vi "Load Zoom FOV table.vi"(8 "error in":errorcluster, 10 "Max Zoom":i32) -> (0 "error out":errorcluster, 2 "FOVs":dbl[][](array[numeric]))   [LabVIEW 2012, in "Sciscan Scope Daemon.lvlib"]
uses:
  Sciscan Scope Daemon.lvlib
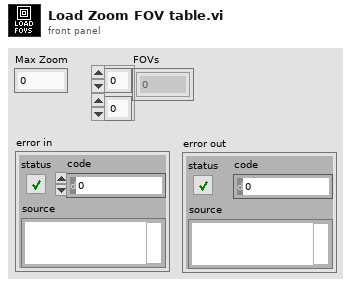
[diagram p1: front panel]
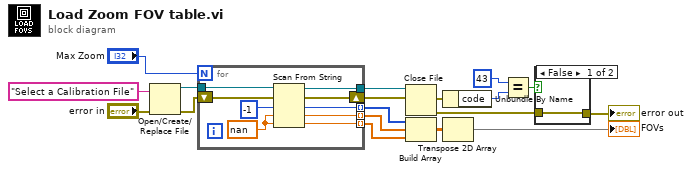
[diagram p0: block diagram]
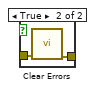
[diagram p2: hidden frame]
diagram:
  n1 = Open/Create/Replace File(error in="error in", prompt="Select a Calibration File") -> (refnum out=w17:refnum<file>, error out=w15:errorcluster)  [unwired: 4 in, 1 out]
  n2 = for {
    N: "Max Zoom" -> [_]
    tunnel: w17 -> [w26]
    tunnel: [w23] -> w16
    shift-right: [w21] -> w14
    shift-left: w15 -> [w22]
    tunnel: [w20] -> w13 mode=indexing
    tunnel: [w19] -> w12 mode=indexing
    tunnel: [w18] -> w9 mode=indexing
    w24 = nan ("input 3")
    n3 = Scan From String(w26, w22, default 1=-1, default 2=w24, default 3=w24) -> (w23:refnum<file>, w21:errorcluster, output 1=w18:i32, output 2=w19:dbl, output 3=w20:dbl)  [unwired: 1 in]
  }
  n4 = Close File(refnum=w16, error in=w14) -> (error out=w2:errorcluster)  [unwired: 1 out]
  n5 = Build Array(w9, w12, w13) -> (w11:dbl[][])
  n6 = Unbundle By Name(w2) -> ("code"=w6:i32)
  n7 = Transpose 2D Array(2D array=w11) -> (transposed array=→"FOVs":dbl[][])
  n8 = Equal?(x=43 ("y"), y=w6) -> (x = y?=w4:bool)
  n9 = case shown="False" w4 {
    tunnel: [w27 w29] -> w3
    tunnel: w2 -> [w27 w28]
    frame False {
    }
    frame True {
      n10 = call <vilib>:"Clear Errors.vi"("error in (no error)"=w28) -> ("error out"=w29:errorcluster)  [unwired: 6 in]
    }
  }
  "error out" <- w3
